vi "JGE2.vi"() -> ()   [LabVIEW 2019]
doc: "This vi produces a pulse width modulation and you can find power output at various points in time"
panel:
  out "Time array":i32[](array[numeric])
  out "Boolean":bool
  out "PW OUT":dbl
  in  "Time input":dbl=1750.0
  in  "Timing control":i32=51
  out "?":cluster{"Array":i32[], dbl[]}(graph)
  out "ramp step":dbl=1.0
  in  "stop":bool
  out "N points":i32=51
  out "PWM array":dbl[](array[numeric])=[30.0, 31.0, 32.0, 33.0, 34.0, 35.0, 36.0, 37.0, 38.0, 39.0, 40.0, 41.0, 42.0, 43.0, 44.0, 45.0, 46.0, 47.0, 48.0, 49.0, 50.0, 50.0, 50.0, 50.0, 50.0, 50.0, 50.0, 50.0, 50.0, 50.0, 50.0, 49.0, 48.0, 47.0, 46.0, 45.0, 44.0, 43.0, 42.0, 41.0, 40.0, 39.0, 38.0, 37.0, 36.0, 35.0, 34.0, 33.0, 32.0, 31.0, 30.0]
  in  "N intervals hold":i32=10
  in  "N intervals ramp":i32=20
  in  "hold PW (us)":dbl=1750.0
  in  "start PW (us)":dbl=1050.0
  # "Speed Control"
  # "Time input (s)"
  # "Juan Gamez\nP3600\nEP2"
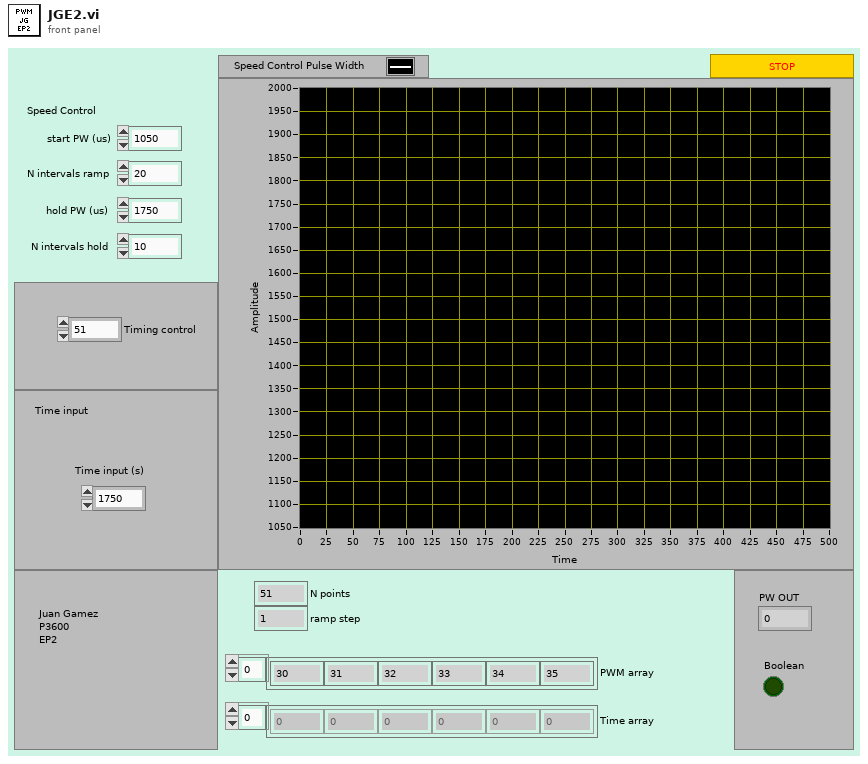
[diagram p1: front panel]
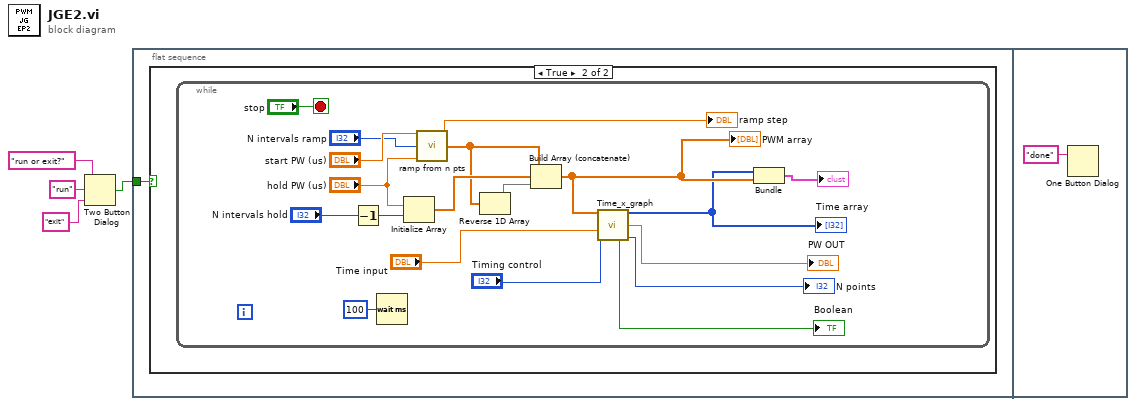
[diagram p0: block diagram]
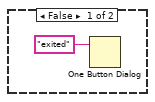
[diagram p2: hidden frame]
diagram:
  n1 = Two Button Dialog(message="run or exit?", 1:"exit" ("F button name (\"Cancel\")"), 2:"run" ("T button name (\"OK\")")) -> (T button?=w1:bool)
  n2 = flat-sequence {
    tunnel: w1 -> [w5]
    frame #0 {
      n3 = case shown="True" w5 {
        frame False {
          n4 = One Button Dialog(message="exited" ("button name (\"OK\")")) -> ()  [unwired: 1 in, 1 out]
        }
        frame True {
          n5 = while {
            stop <- "stop" stop-if-true
            n6 = Decrement(x="N intervals hold") -> (x-1=w15:i32)
            n7 = Wait (ms)(milliseconds to wait=u32 100) -> ()  [unwired: 1 out]
            n8 = Initialize Array("hold PW (us)", w15) -> (w23:dbl[])
            n9 = call "ramp from n pts.vi"("start value"="start PW (us)", "N intervals"="N intervals ramp", "end value"="hold PW (us)") -> ("ramp step"=→"ramp step":dbl, "Values array"=w22:dbl[])  [unwired: 10 in, 1 out]
            n10 = Reverse 1D Array(array=w22) -> (reversed array=w21:dbl[])
            n11 = Build Array (concatenate)(w22, w23, w21) -> (w13:dbl[])
            "PWM array" <- w13
            n12 = call "Time_x_graph.vi"("Inital array"=w13, "Time inputs"="Time input", "Timing control"="Timing control") -> ("Array"=w10:i32[], "PW OUT"=→"PW OUT":dbl, "Boolean 2"=→"Boolean":bool, "N points"=→"N points":i32)  [unwired: 9 in]
            "Time array" <- w10
            n13 = Bundle("Array"=w10, w13) -> (→"?":cluster{"Array":i32[], dbl[]})  [unwired: 1 in]
          }
        }
      }
    }
    frame #1 {
      n14 = One Button Dialog(message="done" ("button name (\"OK\")")) -> ()  [unwired: 1 in, 1 out]
    }
  }
